vi "SendUDP.vi"(7 "data in":string, 8 "error in (no error)":errorcluster, 9 "address":u32, 10 "port or service name":u16, 11 "connection ID":refnum<k16>) -> (0 "error out":errorcluster, 1 "ACK":bool, 2 "data out":string, 3 "connection ID out":refnum<k16>, 4 "NAK":bool, 6 "ERR":bool)   [LabVIEW 2019, in "FPGA.lvlib"]
uses:
  FPGA.lvlib
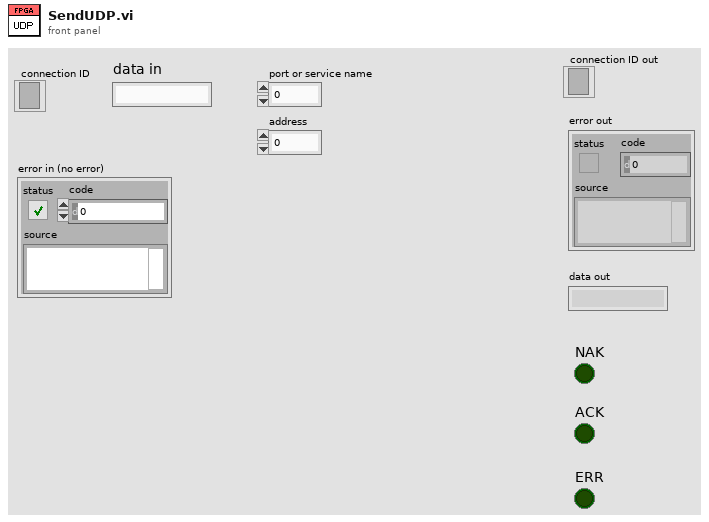
[diagram p1: front panel]
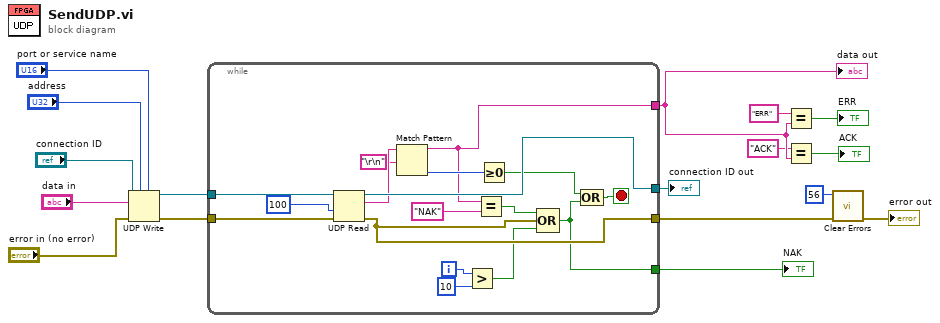
[diagram p0: block diagram]
diagram:
  n1 = UDP Write(address="address", port or service name="port or service name", connection ID="connection ID", data in="data in", 8:"error in (no error)") -> (error out=w8:errorcluster, 3:w7:refnum<k16>)  [unwired: 1 in]
  n2 = while {
    tunnel: w7 -> [w34]
    tunnel: w8 -> [w33]
    tunnel: [w31] -> w1
    tunnel: [w27] -> w10
    tunnel: [w23] -> w9
    tunnel: [w18] -> w15
    i -> [w26]
    stop <- w29 stop-if-true
    n3 = UDP Read(connection ID=w34, timeout ms (25000)=100, 8:w33) -> (data out=w22:string, error out=w27:errorcluster, 3:w31:refnum<k16>)  [unwired: 1 in, 2 out]
    n4 = Match Pattern(string=w22, regular expression="\r\n") -> (before substring=w18:string, offset past match=w20:i32)  [unwired: 1 in, 2 out]
    n5 = Greater?(x=w26, y=10) -> (0:w24:bool)
    n6 = Equal?(x=w18, y="NAK" ("name")) -> (x = y?=w28:bool)
    n7 = Greater Or Equal To 0?(x=w20) -> (x >= 0?=w19:bool)
    n8 = Compound Arithmetic op=OR(w28, w27, w24) -> (w23:bool)
    n9 = Compound Arithmetic op=OR(w19, w23) -> (w29:bool)
  }
  "NAK" <- w9
  "data out" <- w15
  "connection ID out" <- w1
  n10 = Equal?(x="ERR" ("name"), y=w15) -> (x = y?=→"ERR":bool)
  n11 = Equal?(x="ACK" ("name"), y=w15) -> (x = y?=→"ACK":bool)
  n12 = call <vilib>:"Clear Errors.vi"("error in (no error)"=w10, "specific error code to clear (0: all)"=56) -> ("error out"=→"error out":errorcluster)  [unwired: 4 in, 1 out]
